vi "NumberMatchMarcoGonzalez.vi"() -> ()   [LabVIEW 2012]
doc: "The VI goes through the numbers in a given range until it finds the number inputed by the user."
panel:
  out "Number Found":dbl
  in  "0 to:":dbl
  out "# of Guesses":dbl
  in  "Numeric":dbl
  # "Marco Gonzalez\nEA3\n02/28/2017"
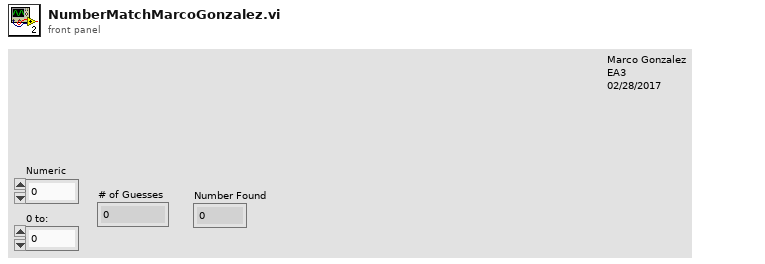
[diagram p1: front panel]
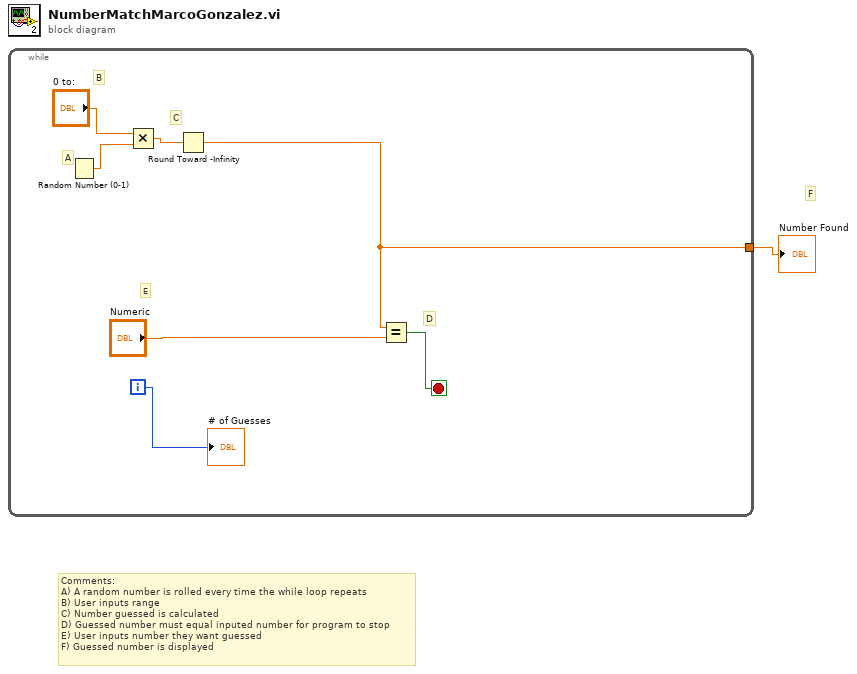
[diagram p0: block diagram]
diagram:
  # "F"
  # "Comments:\nA) A random number is rolled every time the while loop repeats\nB) User inputs range\nC) Number guessed is calculated\nD) Guessed number must equal inputed number for program to stop\nE) User inputs number they want guessed\nF) Guessed number is displayed"
  n1 = while {
    tunnel: [w2] -> w1
    i -> [w8]
    stop <- w6 stop-if-true
    # "E"
    # "D"
    # "C"
    # "B"
    # "A"
    n2 = Random Number (0-1)() -> (number: 0 to 1=w4:dbl)
    n3 = Multiply(x="0 to:", y=w4) -> (x*y=w3:dbl)
    n4 = Round Toward -Infinity(1:w3) -> (0:w2:dbl)
    n5 = Equal?(x=w2, y="Numeric") -> (x = y?=w6:bool)
    "# of Guesses" <- w8
  }
  "Number Found" <- w1
